vi "update images.vi"(7 "intensity plot in":i32[][](array[numeric]), 8 "error in (no error)":errorcluster, 9 "realtime data input":i32[][](array[numeric]), 10 "Energy 2d gate":T1) -> (0 "error out":errorcluster, 1 "Y name":string, 2 "X name":string, 5 "intensity plot out":i32[][](array[numeric]))   [LabVIEW 2016]
doc: "This vi takes the realtime data coming from the pixie 4 and determines which x and y\ncomponents to display. It then sorts them and them to the image to be displayed on\nthe front panel"
uses:
  controls/energy 2d selection.ctl
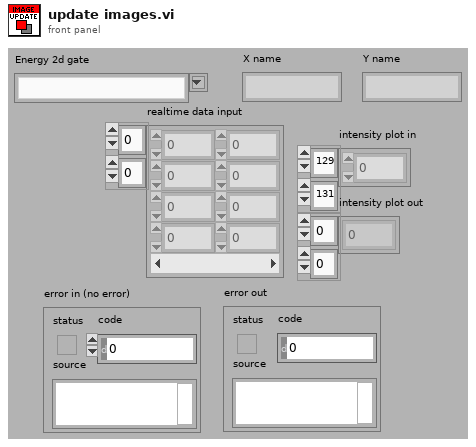
[diagram p1: front panel]
types:
  T1 = typedef "energy 2d selection.ctl" = string
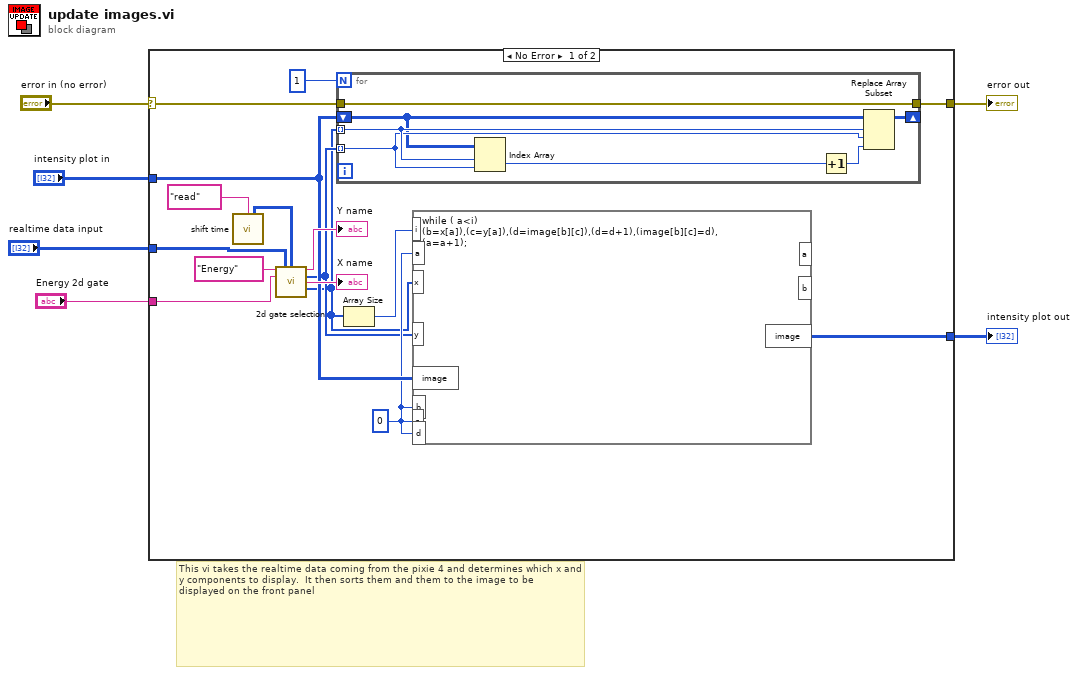
[diagram p0: block diagram]
diagram:
  # "This vi takes the realtime data coming from the pixie 4 and determines which x and y components to display.  It then sorts them and them to the image to be displayed on the front panel"
  n1 = case shown="No Error" "error in (no error)" {
    selector: "error in (no error)" -> [w17 w31]
    tunnel: "realtime data input" -> [w19 _]
    tunnel: [w14 w31] -> w5
    tunnel: "Energy 2d gate" -> [w18 _]
    tunnel: "intensity plot in" -> [w13 w30]
    tunnel: [w10 w30] -> w1
    frame No Error {
      w11 = 0 ("input variable")
      n2 = call "shift time.vi"("shift control"="read") -> ("time array output"=w15:i32[][])  [unwired: 8 in, 6 out]
      n3 = call "2d gate selection.vi"("time or energy"="Energy", "channel 0-4 energy in"=w19, "channel 0-4 time in"=w15, "Energy 2d gate"=w18) -> ("Y name"=→"Y name":string, "Y output array"=w8:i32[], "X name"=→"X name":string, "X output array"=w7:i32[])  [unwired: 5 in, 3 out]
      n4 = for {
        N: 1 -> [_]
        tunnel: w8 -> [w27] mode=indexing
        tunnel: w7 -> [w28] mode=indexing
        tunnel: w17 -> [w23]
        shift-right: [w25] -> _
        shift-left: w13 -> [w24]
        tunnel: [w23] -> w14
        n5 = Index Array(array=w24, index (row)=w28, index (col)=w27) -> (element=w29:i32)
        n6 = Increment(x=w29) -> (x+1=w26:i32)
        n7 = Replace Array Subset(array=w24, new element=w26, index (row)=w28, index (col)=w27) -> (w25:i32[][])
      }
      n8 = Array Size(array=w7) -> (size(s)=w12:i32)
      n9 = formula code="while ( a<i)\n(b=x[a]),(c=y[a]),(d=image[b][c]),(d=d+1),(image[b][c]=d),\n(a=a+1);"("x"=w7, "y"=w8, "image"=w13, "i"=w12, "a"=w11, "b"=w11, "c"=w11, "d"=w11) -> ("image"=w10:i32[][])  [unwired: 2 out]
    }
    frame Error {
    }
  }
  "error out" <- w5
  "intensity plot out" <- w1
